vi "Set Batch Comment.vi"(0 "VISA resource name":refnum<visa-resource-name>, 5 "Comment Number (1)":i32=1 min=1 max=3 format="%.0g", 7 "Comment String (\"\")":string, 11 "error in (no error)":errorcluster) -> (4 "VISA resource name out":refnum<visa-resource-name>, 15 "error out":errorcluster)   [LabVIEW 2020, in "Yokogawa GX Series.lvlib"]
doc: "Sets the batch comment.\n\nCommand: OBatComment"
uses:
  <instrlib>/Yokogawa GX Series/Yokogawa GX Series.lvlib
panel:
  in  "Batch Group Number  (0: OFF)":i32(ring) items=["OFF", "1", "2", "3", "4", "5", "6", "7", "8", "9", "10", "11", "12"]
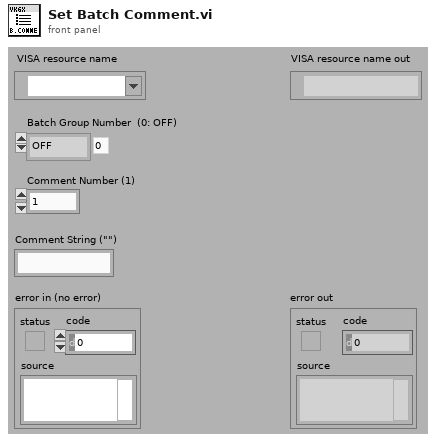
[diagram p1: front panel]
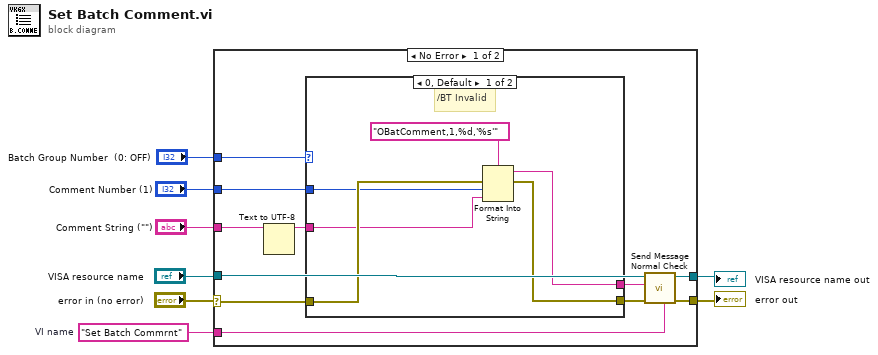
[diagram p0: block diagram]
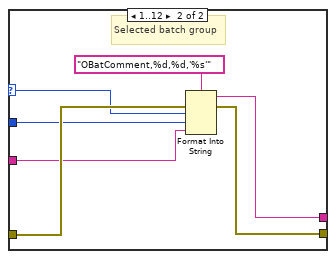
[diagram p2: hidden frame]
diagram:
  w7 = "Set Batch Commrnt"  # VI name
  n1 = case shown="No Error" "error in (no error)" {
    selector: "error in (no error)" -> [w15 w33]
    tunnel: "VISA resource name" -> [w19 w34]
    tunnel: w7 -> [w18 _]
    tunnel: [w17 w34] -> w6
    tunnel: [w16 w33] -> w5
    tunnel: "Comment Number (1)" -> [w11 _]
    tunnel: "Comment String (\"\")" -> [w12 _]
    tunnel: "Batch Group Number  (0: OFF)" -> [w9 _]
    frame No Error {
      n2 = Text to UTF-8(11:w12) -> (3:w10:string)  [unwired: 2 in, 1 out]
      n3 = case shown="0, Default" w9 {
        selector: w9 -> [_ w26]
        tunnel: w15 -> [w24 w31]
        tunnel: [w23 w30] -> w14
        tunnel: [w22 w29] -> w13
        tunnel: w11 -> [w21 w28]
        tunnel: w10 -> [w20 w27]
        frame 0, Default {
          # "/BT Invalid"
          n4 = Format Into String(format string="OBatComment,1,%d,'%s'", error in=w24, w21, w20) -> (resulting string=w22:string, error out=w23:errorcluster)  [unwired: 1 in]
        }
        frame 1..12 {
          # "Selected batch group"
          n5 = Format Into String(format string="OBatComment,%d,%d,'%s'", error in=w31, w26, w28, w27) -> (resulting string=w29:string, error out=w30:errorcluster)  [unwired: 1 in]
        }
      }
      n6 = call <instrlib>:"Send Message Normal Check.vi"("Source (\"\")"=w18, "error in (no error)"=w14, "Send Message (\"\")"=w13, "VISA resource name"=w19) -> ("error out"=w16:errorcluster, "VISA resource name out"=w17:refnum<visa-resource-name>)  [unwired: 2 in, 4 out]
    }
    frame Error {
    }
  }
  "error out" <- w5
  "VISA resource name out" <- w6
